vi "Stop Core.vi"(10 "final error code":i32, 11 "Car Wash CLA - Tom Fantasia in":refnum<class "Car Wash Controller.lvclass">) -> (3 "Car Wash CLA - Tom Fantasia out":refnum<class "Car Wash Controller.lvclass">)   [LabVIEW 2012, in "Car Wash Controller.lvlib" / "Car Wash Controller.lvclass"]
uses:
  Car Wash Controller.lvclass
  <vilib>/ActorFramework/Actor/Actor.lvclass
  <vilib>/ActorFramework/Stop Msg/Stop Msg.lvclass
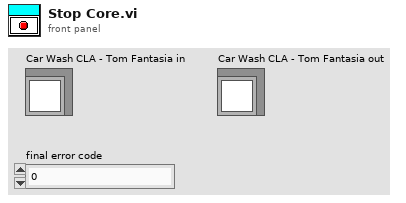
[diagram p1: front panel]
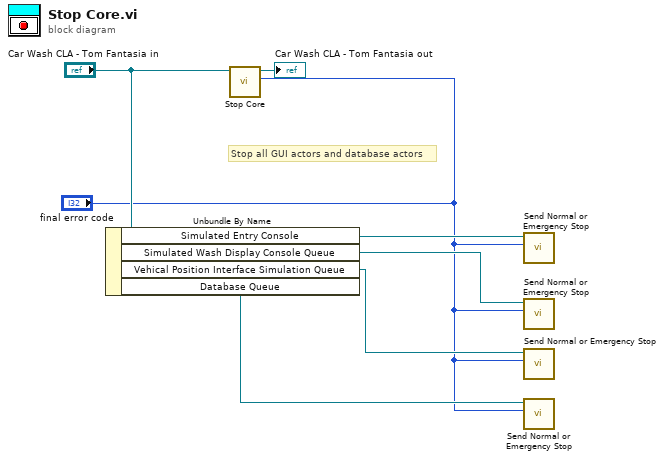
[diagram p0: block diagram]
diagram:
  # "Stop all GUI actors and database actors"
  n1 = Unbundle By Name("Car Wash CLA - Tom Fantasia in") -> ("Simulated Entry Console"=w5:refnum<class "Message Enqueuer.lvclass">, "Simulated Wash Display Console Queue"=w4:refnum<class "Message Enqueuer.lvclass">, "Vehical Position Interface Simulation Queue"=w3:refnum<class "Message Enqueuer.lvclass">, "Database Queue"=w2:refnum<class "Message Enqueuer.lvclass">)
  n2 = call-parent "Stop Core.vi"("final error code"="final error code", "Actor in"="Car Wash CLA - Tom Fantasia in") -> ("Actor out"=→"Car Wash CLA - Tom Fantasia out":refnum<class "Car Wash Controller.lvclass">)  [unwired: 9 in]
  n3 = call <vilib>:"Send Normal or Emergency Stop.vi"("final error code"="final error code", "Message Enqueuer"=w5) -> ()  [unwired: 9 in, 1 out]
  n4 = call <vilib>:"Send Normal or Emergency Stop.vi"("final error code"="final error code", "Message Enqueuer"=w4) -> ()  [unwired: 9 in, 1 out]
  n5 = call <vilib>:"Send Normal or Emergency Stop.vi"("final error code"="final error code", "Message Enqueuer"=w3) -> ()  [unwired: 9 in, 1 out]
  n6 = call <vilib>:"Send Normal or Emergency Stop.vi"("final error code"="final error code", "Message Enqueuer"=w2) -> ()  [unwired: 9 in, 1 out]
